vi "In-Line-Pressure 2016.vi"(6 "Zero Pressure\n(F = leave as is)":bool=TRUE, 9 "In-Line Pressure Slope":dbl=47.84 format="%.2f", 10 "Sensor Voltages Cluster":T1, 11 "In-Line Pressure Offset":dbl=40.0 format="%.2f") -> (3 "Pressure":dbl=0.003808000000006473 format="%.2f")   [LabVIEW 2016]
uses:
  controls/MCC DAQ Readings.ctl
panel:
  out "Voltage":dbl=0.8362 format="%.3f"
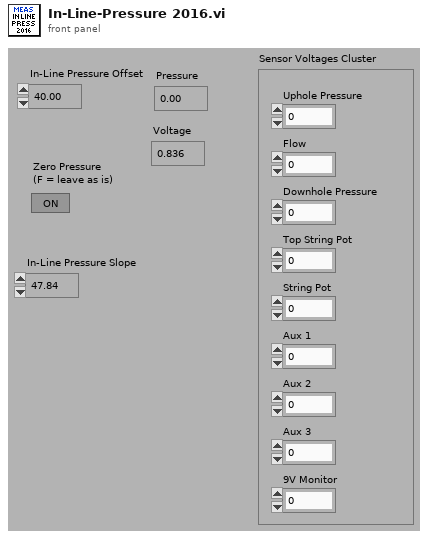
[diagram p1: front panel]
types:
  T1 = typedef "MCC DAQ Readings.ctl" = cluster{"Uphole Pressure":dbl, "Flow":dbl, "Downhole Pressure":dbl, "Top String Pot":dbl, "String Pot":dbl, "Aux 1":dbl, "Aux 2":dbl, "Aux 3":dbl, "9V Monitor":dbl}
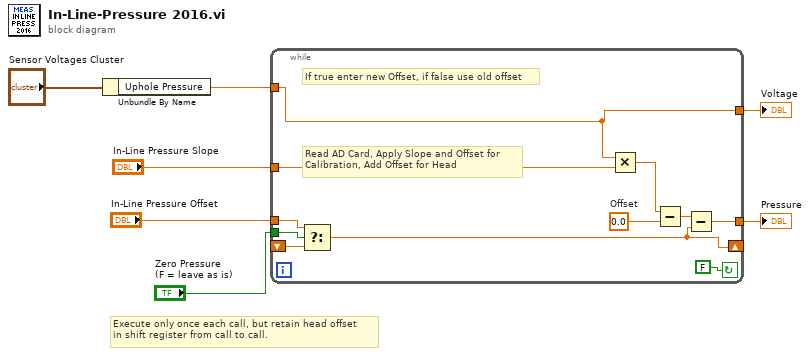
[diagram p0: block diagram]
diagram:
  # "Execute only once each call, but retain head offset \nin shift register from call to call."
  n1 = Unbundle By Name("Sensor Voltages Cluster") -> ("Uphole Pressure"=w1:dbl)
  n2 = while {
    tunnel: "Zero Pressure\n(F = leave as is)" -> [w14]
    tunnel: "In-Line Pressure Offset" -> [w15]
    shift-left: _ -> [w16]
    shift-right: [w10] -> _
    tunnel: [w13] -> w7
    tunnel: "In-Line Pressure Slope" -> [w9]
    tunnel: [w8] -> w3
    tunnel: w1 -> [w8]
    stop <- FALSE continue-if-true
    w17 = 0.0  # Offset
    # "Read AD Card, Apply Slope and Offset for\nCalibration, Add Offset for Head"
    # "If true enter new Offset, if false use old offset"
    n3 = Select(t=w15, s=w14, f=w16) -> (s? t:f=w10:dbl)
    n4 = Multiply(x=w8, y=w9) -> (x*y=w18:dbl)
    n5 = Subtract(x=w18, y=w17) -> (x-y=w11:dbl)
    n6 = Subtract(x=w11, y=w10) -> (x-y=w13:dbl)
  }
  "Pressure" <- w7
  "Voltage" <- w3
